vi "Close.vi"(8 "error in (no error)":errorcluster, 11 "XNET Base CFG in":refnum<class "XNET Base CFG.lvclass">) -> (0 "error out":errorcluster, 3 "XNET Base CFG out":refnum<class "XNET Base CFG.lvclass">)   [LabVIEW 2024, in "XNET Base CFG.lvclass"]
uses:
  XNET Base CFG.lvclass
  XNET Base CFG.lvclass/XNET Base CFG.ctl
  Configurations/CFG JSON/CFG JSON.lvclass
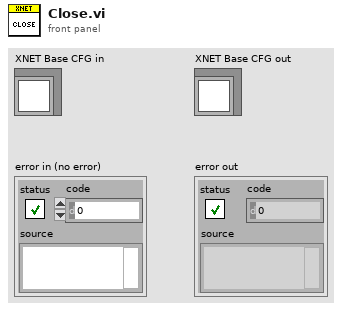
[diagram p1: front panel]
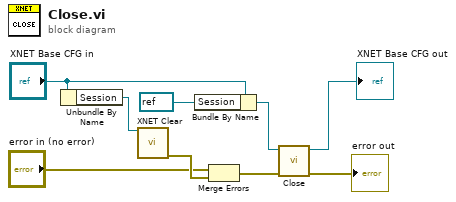
[diagram p0: block diagram]
diagram:
  n1 = Unbundle By Name("XNET Base CFG in") -> ("Session"=w8:refnum<k21>)
  n2 = call <vilib>:"XNET Clear.vi"("session in"=w8) -> ("error out"=w9:errorcluster)  [unwired: 14 in]
  n3 = Bundle By Name(cluster="XNET Base CFG in", "Session"=refnum<k21> refnum ("session")) -> (w2:refnum<class "XNET Base CFG.lvclass">)
  n4 = Merge Errors("error in (no error)", w9) -> (w5:errorcluster)
  n5 = call-parent "Close.vi"("error in"=w5, "CFG Base in"=w2) -> ("error out"=→"error out":errorcluster, "CFG Base out"=→"XNET Base CFG out":refnum<class "XNET Base CFG.lvclass">)  [unwired: 8 in]
